vi "PythonAnalyze.vi"(8 "error in (no error)":errorcluster, 9 "Python Session In":refnum<k35>, 10 "Frame Space":T2, 11 "Cam Session":T1) -> (0 "Python session out 2":refnum<k35>, 1 "Cam Session Out 2":T1, 2 "Mask":bool, 3 "Image Out":T2(plugin-control), 4 "error out":errorcluster)   [LabVIEW 2020]
doc: "This VI uses IMAQ library and Python connectivity tools to acquire an image, analyze it and finally return it in an output."
uses:
  <vilib>/userdefined/High Color/IMAQdx.ctl
  <vilib>/vision/Image Controls.llb/IMAQ Image.ctl
  <vilib>/vision/NI_Vision_Development_Module.lvlib
  <vilib>/vision/driver/NI_Vision_Acquisition_Software.lvlib
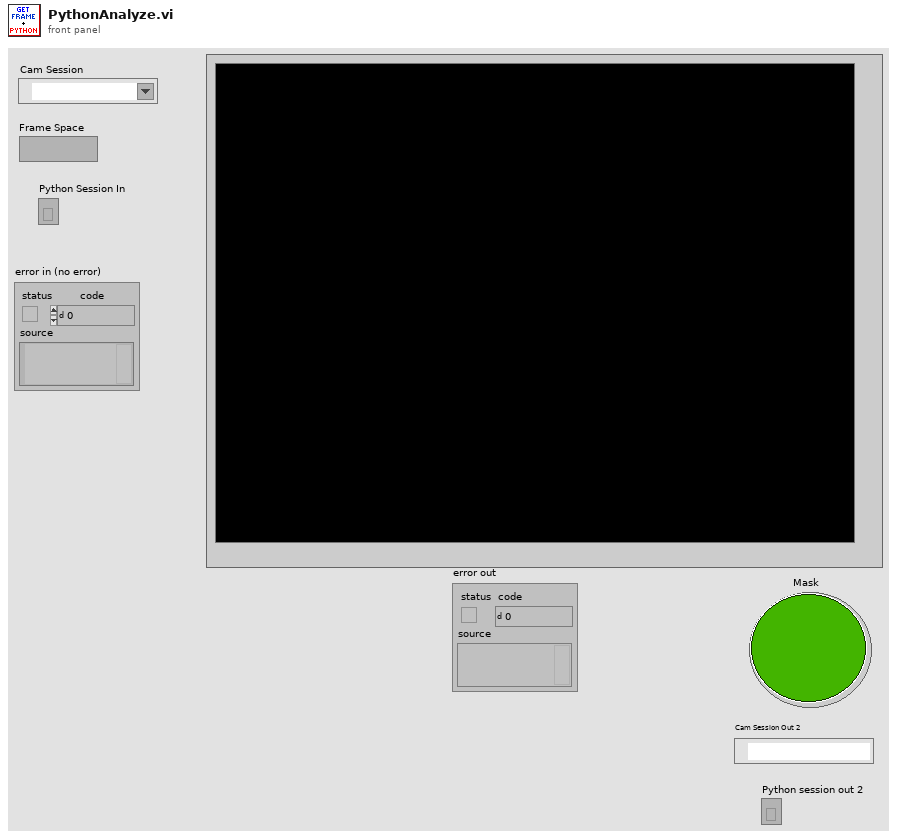
[diagram p1: front panel]
types:
  T1 = typedef "IMAQdx.ctl" = refnum<k21>
  T2 = typedef "IMAQ Image.ctl" = refnum<image>
  T3 = typedef "Image Type" = u32
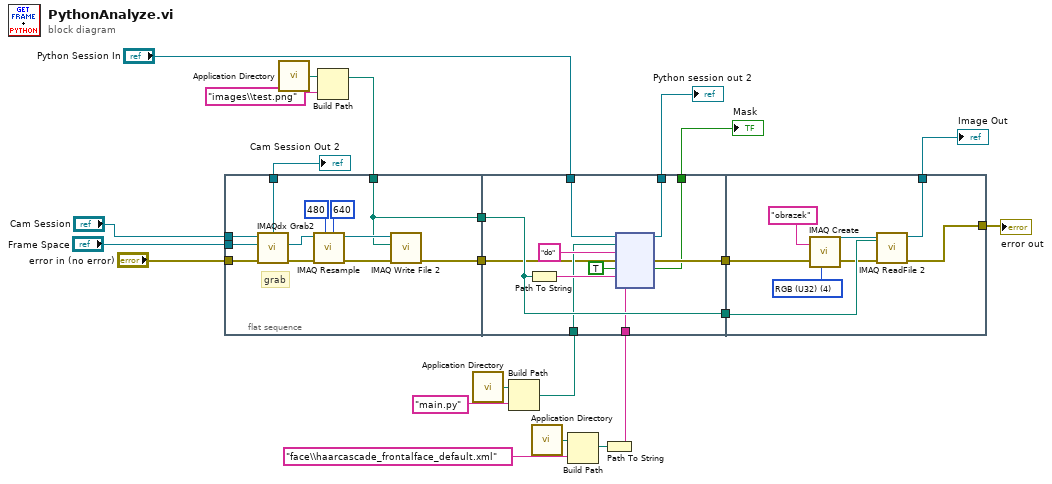
[diagram p0: block diagram]
diagram:
  n1 = flat-sequence {
    tunnel: [w24] -> w13
    tunnel: "Cam Session" -> [w33]
    tunnel: "Frame Space" -> [w32]
    tunnel: [w31] -> w7
    tunnel: w19 -> [w24]
    tunnel: "error in (no error)" -> [w30]
    tunnel: [w27] -> w12
    tunnel: w13 -> [w44]
    tunnel: [w44] -> w11
    tunnel: [w43] -> w6
    tunnel: w18 -> [w42]
    tunnel: w12 -> [w41]
    tunnel: [w40] -> w10
    tunnel: w14 -> [w38]
    tunnel: "Python Session In" -> [w37]
    tunnel: [w36] -> w2
    tunnel: w11 -> [w54]
    tunnel: w10 -> [w49]
    tunnel: [w53] -> w5
    tunnel: [w47] -> w1
    frame #0 {
      # "grab"
      n2 = call <vilib>:"IMAQdx Grab2.vi"("error in"=w30, "Image In"=w32, "Session In"=w33) -> ("error out"=w29:errorcluster, "Image Out"=w26:T2, "Session Out"=w31:T1)  [unwired: 5 in, 1 out]
      n3 = call "IMAQ Resample"("X Resolution"=640, "Y Resolution"=480, "error in (no error)"=w29, "Image Src"=w26) -> ("error out"=w28:errorcluster, "Image Dst Out"=w25:T2)  [unwired: 6 in]
      n4 = call-poly "IMAQ Write File 2"("error in (no error)"=w28, "File Path"=w24, "Image"=w25) -> ("error out"=w27:errorcluster)  [unwired: 7 in, 1 out]
    }
    frame #1 {
      n5 = Path To String(path=w44) -> (string=w45:string)
      n6 = node ("Python Node")(w37, w42, "do" ("function name"), w41, TRUE ("Maska"), w45, w38) -> (w43:refnum<k35>, w40:errorcluster, w36:bool)  [unwired: 2 in, 2 out]
    }
    frame #2 {
      w51 = T3 4 items=["Grayscale (U8)", "Grayscale (I16)", "Grayscale (SGL)", "Complex (CSG)", "RGB (U32)", "HSL (U32)", "RGB (U64)", "Grayscale (U16)"] ("Image Type")
      n7 = call "IMAQ Create"("Image Name"="obrazek", "Image Type"=w51, "error in (no error)"=w49) -> ("New Image"=w50:T2, "error out"=w48:errorcluster)  [unwired: 2 in]
      n8 = call "IMAQ ReadFile 2"("File Path"=w54, "error in (no error)"=w48, "Image"=w50) -> ("error out"=w53:errorcluster, "Image Out"=w47:T2)  [unwired: 4 in, 3 out]
    }
  }
  n9 = call <vilib>:"Application Directory.vi"() -> ("Application Directory"=w23:path)
  n10 = Build Path(base path=w23, name or relative path="images\\test.png") -> (appended path=w19:path)
  n11 = call <vilib>:"Application Directory.vi"() -> ("Application Directory"=w21:path)
  n12 = Build Path(base path=w21, name or relative path="main.py") -> (appended path=w18:path)
  n13 = call <vilib>:"Application Directory.vi"() -> ("Application Directory"=w17:path)
  n14 = Build Path(base path=w17, name or relative path="face\\haarcascade_frontalface_default.xml") -> (appended path=w15:path)
  n15 = Path To String(path=w15) -> (string=w14:string)
  "Cam Session Out 2" <- w7
  "Python session out 2" <- w6
  "error out" <- w5
  "Mask" <- w2
  "Image Out" <- w1
